vi "GetBroadcast.vi"(8 "Error In":errorcluster[](array[cluster]), 9 "BdcstInfo":variant, 11 "clBusData In":T2={"BusNumber"=0, "EvtPluginINIFilePath"=path "", "EvtParams"=[], "EvtConfig"={"UTC Time 0"=timestamp(0 s since 1904-01-01), "Nominal Frequency"=60, "Reporting Rate"=60, "Fsamp"=960, "PosSeq"=FALSE}, "Start Time"=0.0, "End Time"=0.0, "PmuImpairPluginINIFilePath"=path "", "PmuImpairParams "=[["960"], ["8.19"], ["164"]], "PmuImpairConfig"={"FilterType"="", "bPosSeq"=TRUE}, "NetImpPluginINIFilePath"=path "", "NetImpParams"=[], "FlagImpPluginINIFilePath"=path "", "FlagImpParams"=[], "EvtReportArray"=[], "EventSignalArray"=[], "ImpairReportArray"=[], "NetworkTime"=[], "PktLoss"=[], "FlagImpArray"=[], "OutputToFilePluginINIFilePath"=path "", "Output File Path"=path "", "clConfigOptions"={"TIME_BASE"=1000000, "STN"="Bus_1", "IDCODE"=0, "rdoPolRect"=enum."Rectangular", "rdoFloatInt"=enum."Float", "PHUNIT"=1000000, "rdoFreqDfreq"=enum."Float", "CHNAM"=["VA", "VB", "VC", "V+", "IA", "IB", "IC", "I+"], "chkCfg2Prefix"=TRUE}, "AppPluginINIFilePath"=path "", "AppConfig"=variant, "AppOutput"=variant} {"clConfigOptions"."PHUNIT" max=16777216 step=1 format="%08d"; "clConfigOptions"."IDCODE" format="%02x"; "clConfigOptions"."TIME_BASE" max=16777216 step=1 format="%08d"; "ImpairReportArray"."Synx" format="%#_4g"; "EvtReportArray"."Synx" format="%#_4g"; "EvtConfig"."Reporting Rate" items=["10 FPS"=10, "12 FPS"=12, "15 FPS"=15, "20 FPS"=20, "25 FPS"=25, "30 FPS"=30, "50 FPS"=50, "60 FPS"=60]; "EvtConfig"."Nominal Frequency" items=["50 Hz"=50, "60 Hz"=60]}) -> (0 "Error Out":errorcluster[](array[cluster]), 3 "clBusData Out":T2={"BusNumber"=0, "EvtPluginINIFilePath"=path "", "EvtParams"=[], "EvtConfig"={"UTC Time 0"=timestamp(0 s since 1904-01-01), "Nominal Frequency"=60, "Reporting Rate"=60, "Fsamp"=960, "PosSeq"=FALSE}, "Start Time"=0.0, "End Time"=0.0, "PmuImpairPluginINIFilePath"=path "", "PmuImpairParams "=[["960"], ["8.19"], ["164"]], "PmuImpairConfig"={"FilterType"="", "bPosSeq"=TRUE}, "NetImpPluginINIFilePath"=path "", "NetImpParams"=[], "FlagImpPluginINIFilePath"=path "", "FlagImpParams"=[], "EvtReportArray"=[], "EventSignalArray"=[], "ImpairReportArray"=[], "NetworkTime"=[], "PktLoss"=[], "FlagImpArray"=[], "OutputToFilePluginINIFilePath"=path "", "Output File Path"=path "", "clConfigOptions"={"TIME_BASE"=1000000, "STN"="Bus_1", "IDCODE"=0, "rdoPolRect"=enum."Rectangular", "rdoFloatInt"=enum."Float", "PHUNIT"=1000000, "rdoFreqDfreq"=enum."Float", "CHNAM"=["VA", "VB", "VC", "V+", "IA", "IB", "IC", "I+"], "chkCfg2Prefix"=TRUE}, "AppPluginINIFilePath"=path "", "AppConfig"=variant, "AppOutput"=variant} {"clConfigOptions"."PHUNIT" max=16777216 step=1 format="%08d"; "clConfigOptions"."IDCODE" format="%02x"; "clConfigOptions"."TIME_BASE" max=16777216 step=1 format="%08d"; "ImpairReportArray"."Synx" format="%#_4g"; "EvtReportArray"."Synx" format="%#_4g"; "EvtConfig"."Reporting Rate" items=["10 FPS"=10, "12 FPS"=12, "15 FPS"=15, "20 FPS"=20, "25 FPS"=25, "30 FPS"=30, "50 FPS"=50, "60 FPS"=60]; "EvtConfig"."Nominal Frequency" items=["50 Hz"=50, "60 Hz"=60]})   [LabVIEW 2017, in "Bus_class.lvlib" / "Bus.lvclass"]
uses:
  Bus.lvclass
  Public/TypeDefs/clBusData.ctl
  FrontPanel/TypeDefs/clEventConfig.ctl
  Modules/PmuImpairPlugins/PmuImpairPluginBase_class/TypeDefs/clImpairConfig.ctl
  Modules/EventPlugins/EventPluginBaseClass/TypeDefs/clEvtReportArray.ctl
  Modules/EventPlugins/EventPluginBaseClass/TypeDefs/clEvtReport.ctl
  Modules/EventPlugins/EventPluginBaseClass/TypeDefs/dblEvtSignalArray.ctl
  Modules/NetworkImpairmentModule/PublicAPI/Arguments/Broadcasts/dblNetworkTime.ctl
  Modules/NetworkImpairmentModule/PublicAPI/Arguments/Broadcasts/dblPktLoss.ctl
  Modules/FlagImpairModule/PublicAPI/Arguments/Broadcasts/ui32FlagImpairmentArray.ctl
  Modules/OutputToFilePlugins/OutputToFileBasePlugin/Typedefs/PmuCfgOpt.ctl
  ModuleType.ctl
  BdcstInfo.ctl
  Modules/EventModule/Protected/Broadcasts/clBroadcastEvents.ctl
  Modules/EventModule/Protected/clEventType.ctl
  Modules/EventModule/PublicAPI/Arguments/Broadcasts/clErrorRpt.ctl
  Modules/EventPlugins/EventPluginBaseClass/TypeDefs/clEvtConfig.ctl
  Modules/EventModule/PublicAPI/Arguments/Requests/dblTimeArray.ctl
  Modules/EventModule/PublicAPI/Arguments/Requests/dblEvtParams.ctl
  Modules/PmuImpairModule/Protected/Broadcasts/clBroadcastEvents.ctl
  Modules/PmuImpairModule/Protected/clEventType.ctl
  Modules/NetworkImpairmentModule/Protected/Broadcasts/clBroadcastEvents.ctl
  Modules/NetworkImpairmentModule/Protected/clEventType.ctl
  Modules/FlagImpairModule/Protected/Broadcasts/clBroadcastEvents.ctl
  Modules/FlagImpairModule/Protected/clEventType.ctl
  Modules/AppModule/Protected/Broadcasts/clBroadcastEvents.ctl
  Modules/AppModule/Protected/clEventType.ctl
  Modules/OutputToFileModule/Protected/Broadcasts/clBroadcastEvents.ctl
  Modules/OutputToFileModule/Private/clEventType.ctl
  <vilib>/Utility/error.llb/Error Cluster From Error Code.vi
  <vilib>/ErrorRing/Error Ring.xnode
  <userlib>/NIST/NISTErrorLib/NISTErrorLib.lvlib
  Modules/EventModule/EventModule.lvlib
  Framework.lvlib
  Modules/EventPlugins/EventPluginBaseClass/EventPluginBaseClass.lvclass
  Modules/PmuImpairPlugins/PmuImpairPluginBase_class/PmuImpairPluginBase.lvclass
  Modules/NetworkImpairmentModule/NetworkImpairmentModule.lvlib
  Modules/FlagImpairModule/FlagImpairModule.lvlib
  Modules/AppModule/AppModule.lvlib
  Modules/PmuImpairModule/PmuImpairModule.lvlib
  Modules/OutputToFileModule/OutputToFileModule.lvlib
  Modules/OutputToFilePlugins/OutputToFileBasePlugin/OutputToFileBasePlugin.lvclass
panel:
  out "ModuleType":T1
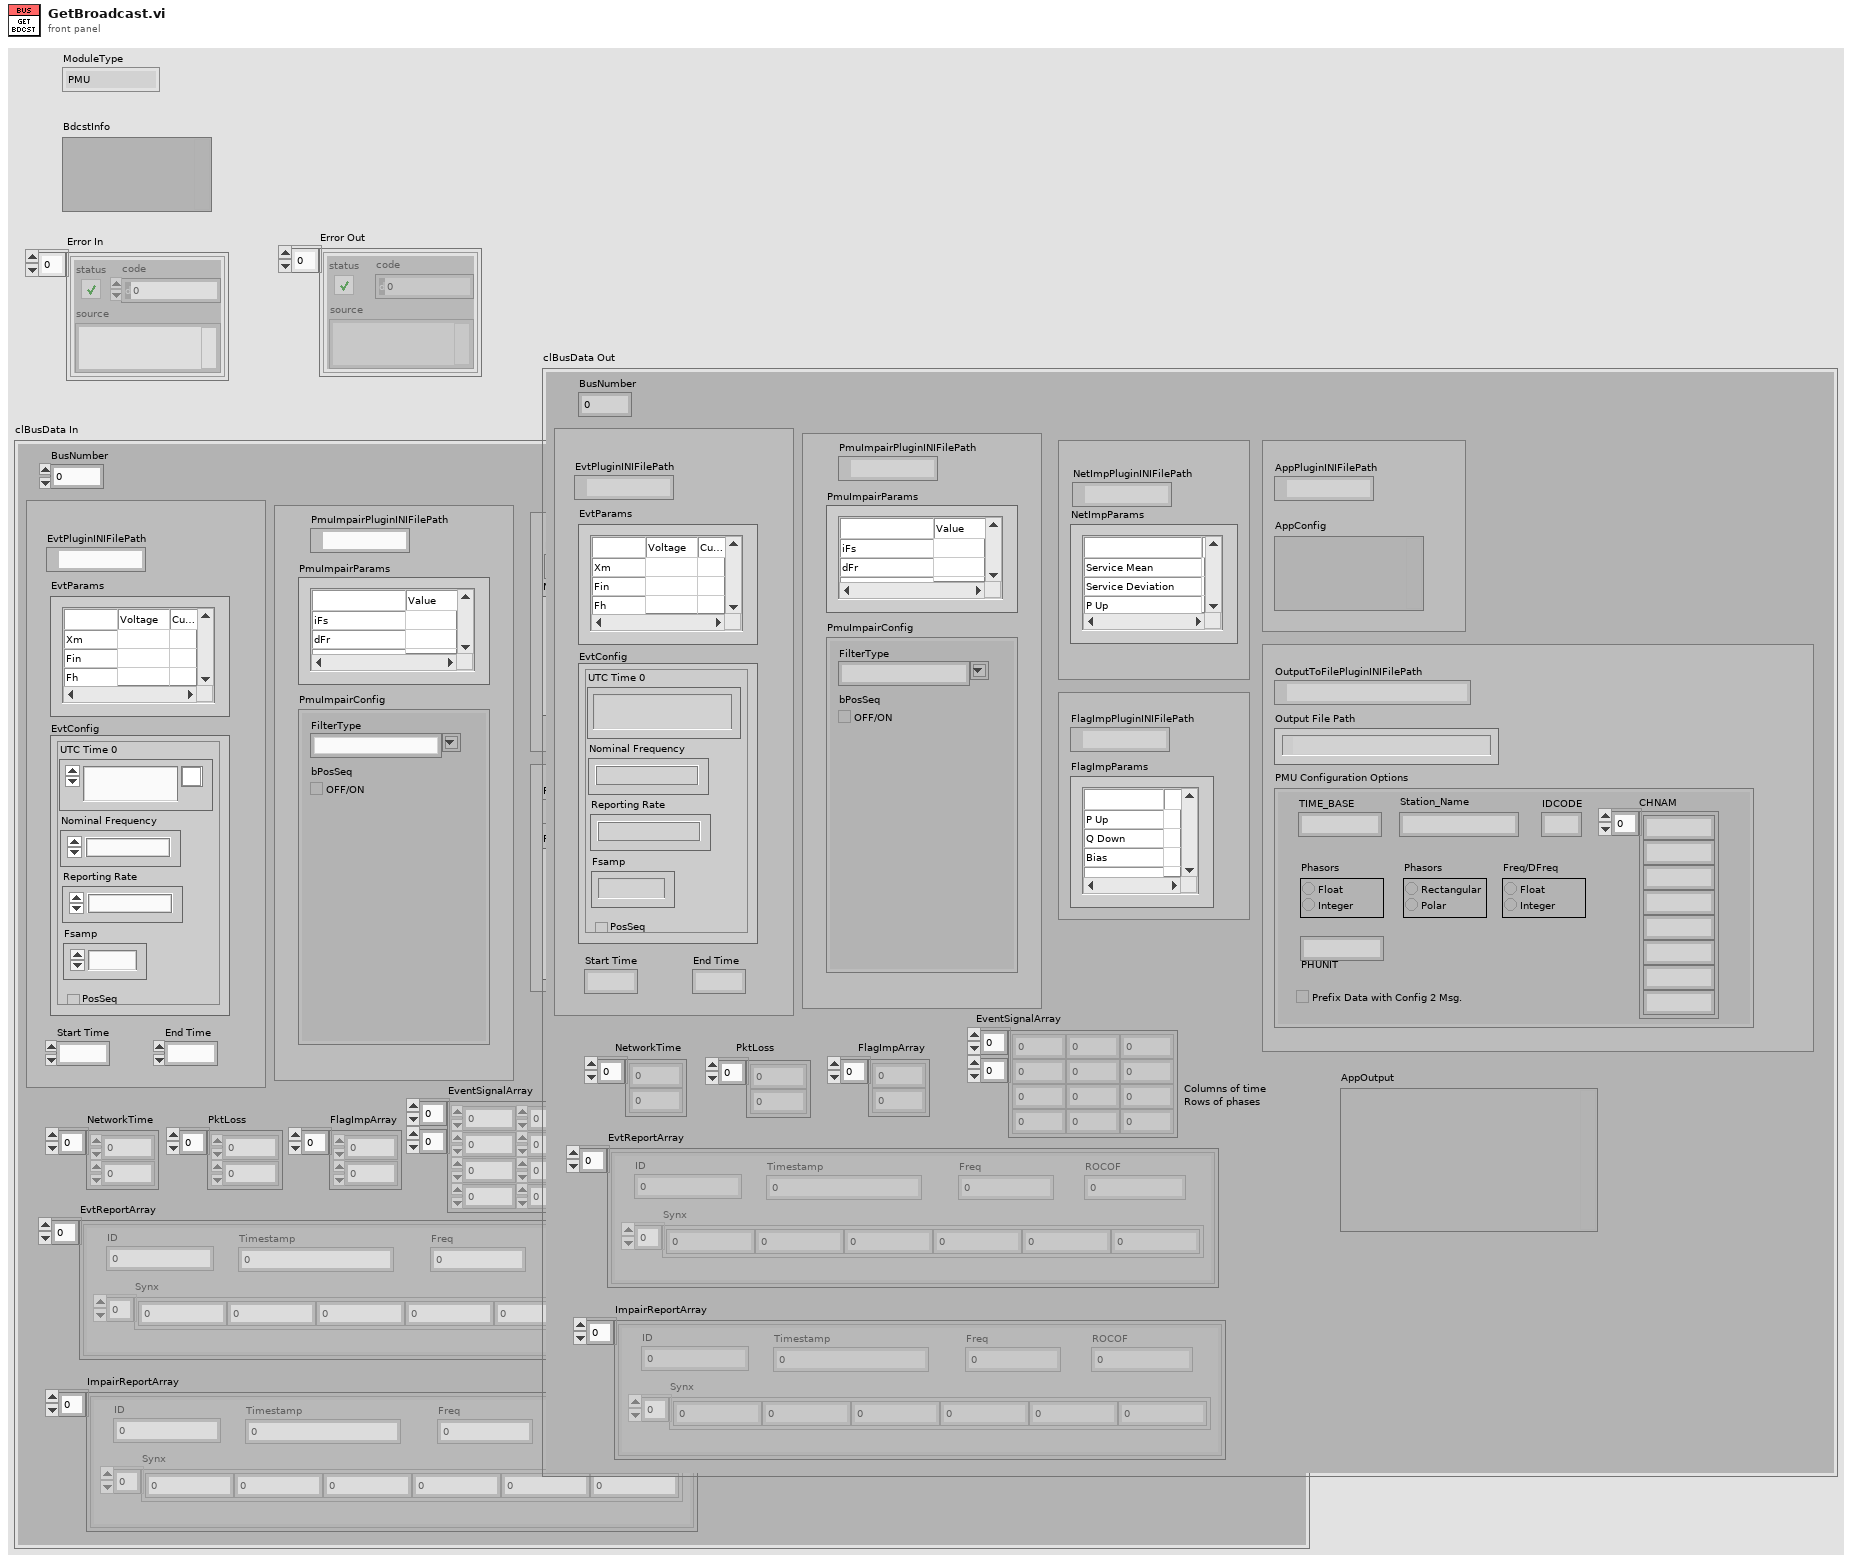
[diagram p1: front panel]
types:
  T1 = typedef "Bus_class.lvlib/Bus.lvclass/ModuleType.ctl" = enum16{"PMU", "Event", "Network", "Flag", "App", "OutToFile"}
  T2 = typedef "Bus_class.lvlib/Bus.lvclass/clBusData.ctl" = cluster{"BusNumber":u8, "EvtPluginINIFilePath":path, "EvtParams":string[][], "EvtConfig":T3, "Start Time":dbl, "End Time":dbl, "PmuImpairPluginINIFilePath":path, "PmuImpairParams ":string[][], "PmuImpairConfig":T4, "NetImpPluginINIFilePath":path, "NetImpParams":string[][], "FlagImpPluginINIFilePath":path, "FlagImpParams":string[][], "EvtReportArray":T5, "EventSignalArray":T7, "ImpairReportArray":T5, "NetworkTime":T8, "PktLoss":T9, "FlagImpArray":T10, "OutputToFilePluginINIFilePath":path, "Output File Path":path, "clConfigOptions":T11, "AppPluginINIFilePath":path, "AppConfig":variant, "AppOutput":variant}
  T3 = typedef "Framework.lvlib/clEventConfig.ctl" = cluster{"UTC Time 0":timestamp, "Nominal Frequency":u16, "Reporting Rate":u16, "Fsamp":u32, "PosSeq":bool}
  T4 = typedef "PmuImpairPlugins.lvlib/PmuImpairPluginBase.lvclass/clImpairConfig.ctl" = cluster{"FilterType":string, "bPosSeq":bool}
  T5 = typedef "EventPlugins.lvlib/EventPluginBaseClass.lvclass/clEvtReportArray.ctl" = T6[]
  T6 = typedef "EventPlugins.lvlib/EventPluginBaseClass.lvclass/clEvtReport.ctl" = cluster{"Timestamp":dbl, "Synx":cdb[], "Freq":dbl, "ROCOF":dbl, "ID":i16}
  T7 = typedef "EventPlugins.lvlib/EventPluginBaseClass.lvclass/dblEvtSignalArray.ctl" = dbl[][]
  T8 = typedef "NetworkImpairmentModule.lvlib/dblNetworkTime.ctl" = dbl[]
  T9 = typedef "NetworkImpairmentModule.lvlib/dblPktLoss.ctl" = dbl[]
  T10 = typedef "FlagImpairModule.lvlib/ui32FlagImpairmentArray.ctl" = u32[]
  T11 = typedef "OutputToFilePlugins.lvlib/OutputToFileBasePlugin.lvclass/PmuCfgOpt.ctl" = cluster{"TIME_BASE":u64, "STN":string, "IDCODE":u16, "rdoPolRect":enum32{"Rectangular", "Polar"}, "rdoFloatInt":enum32{"Float", "Integer"}, "PHUNIT":u64, "rdoFreqDfreq":enum32{"Float", "Integer"}, "CHNAM":string[], "chkCfg2Prefix":bool}
  T12 = typedef "Bus_class.lvlib/Bus.lvclass/BdcstInfo.ctl" = cluster{"ModuleType":T1, "ModuleID":i32, "UsrEvtRef":variant, "ScriptCmd":string}
  T13 = typedef "EventModule.lvlib/clErrorRpt.ctl" = cluster{"error":errorcluster, "AdditionalInfo":string}
  T14 = typedef "EventPlugins.lvlib/EventPluginBaseClass.lvclass/clEvtConfig.ctl" = cluster{"T0(UTC)":dbl, "F0":dbl, "Fs":i32, "FSamp":u32, "bPosSeq":bool}
  T15 = typedef "EventModule.lvlib/dblTimeArray.ctl" = dbl[]
  T16 = typedef "EventModule.lvlib/dblEvtParams.ctl" = dbl[][]
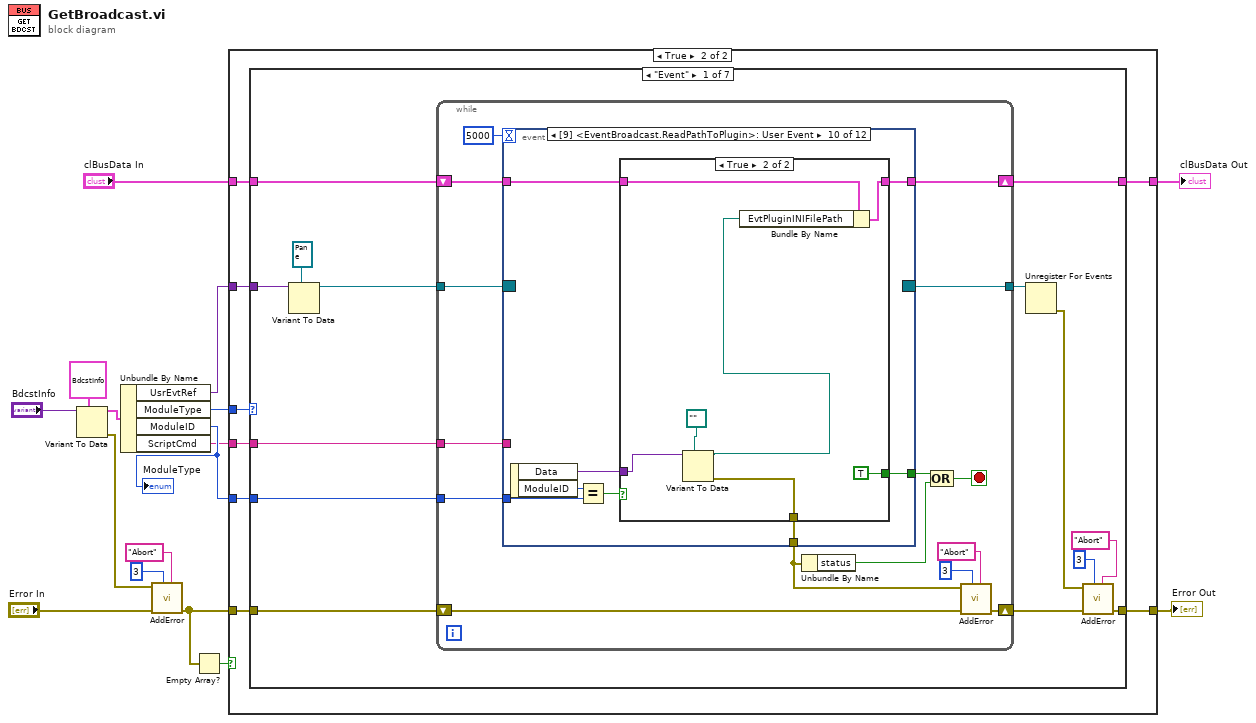
[diagram p0: block diagram]
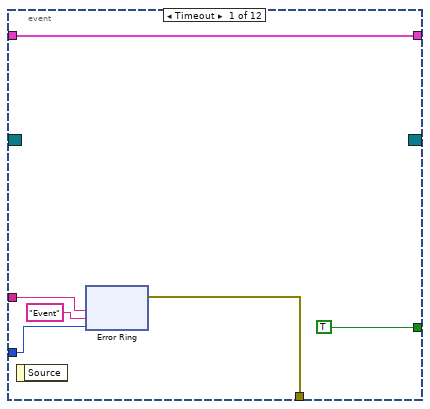
[diagram p3: hidden frame]
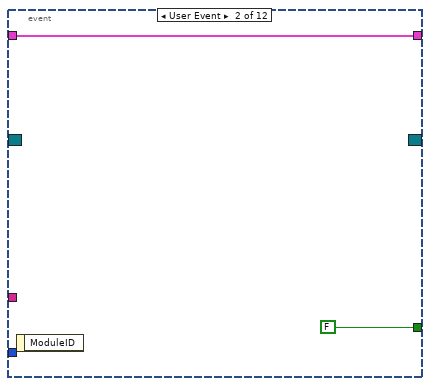
[diagram p4: hidden frame]
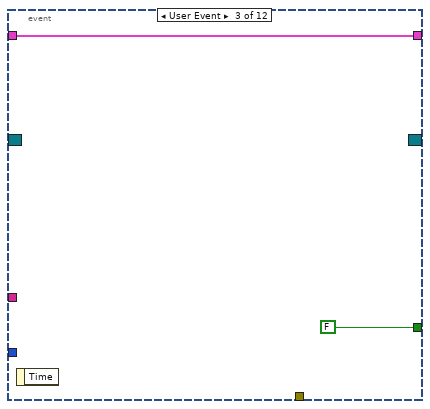
[diagram p5: hidden frame]
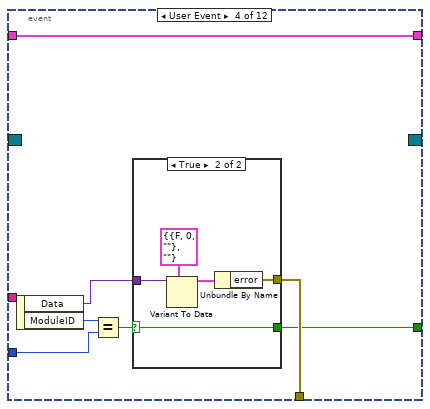
[diagram p6: hidden frame]
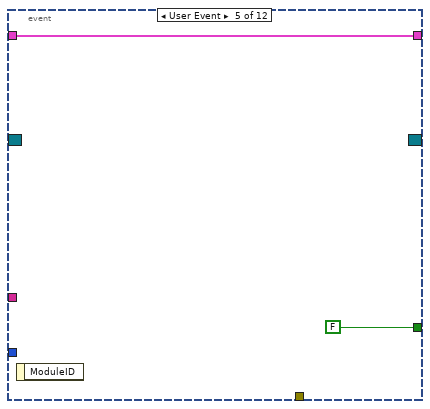
[diagram p8: hidden frame]
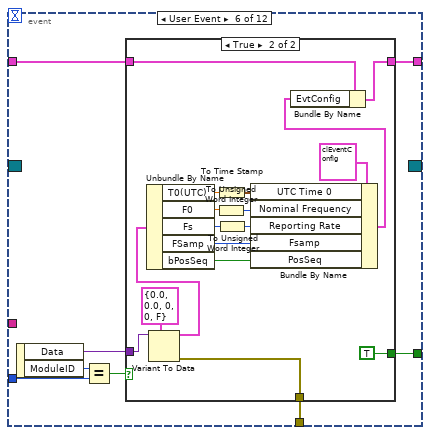
[diagram p9: hidden frame]
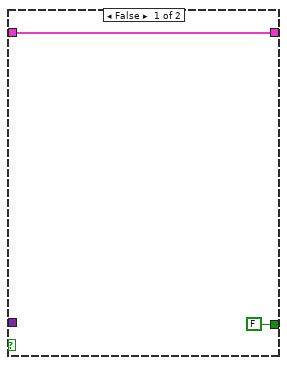
[diagram p10: hidden frame]
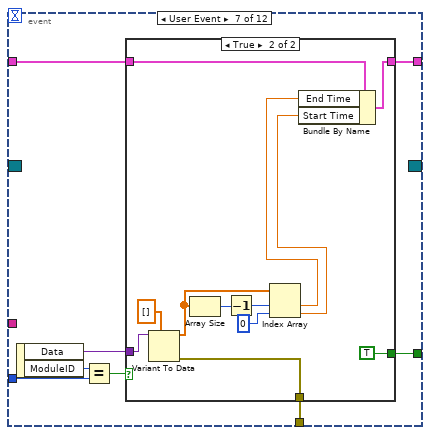
[diagram p11: hidden frame]
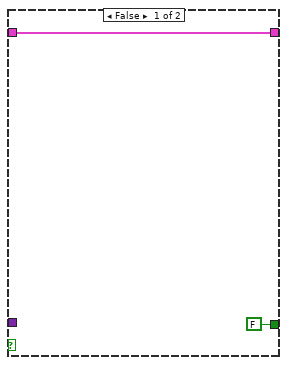
[diagram p12: hidden frame]
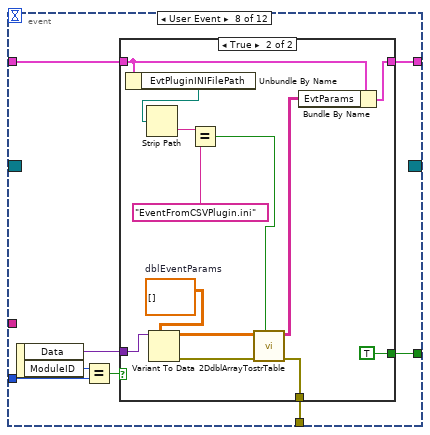
[diagram p13: hidden frame]
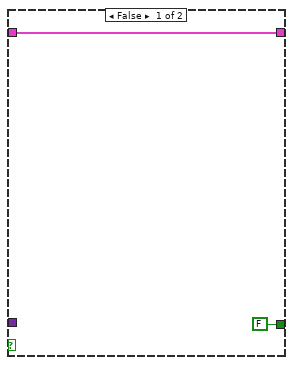
[diagram p14: hidden frame]
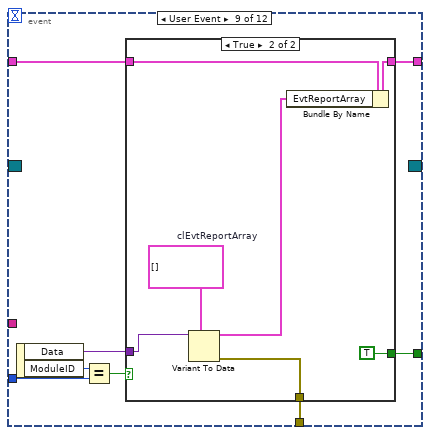
[diagram p15: hidden frame]
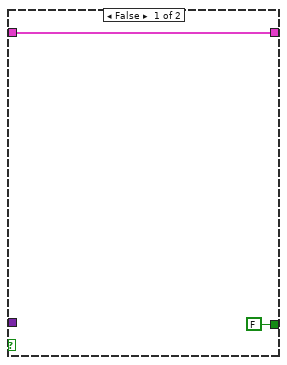
[diagram p16: hidden frame]
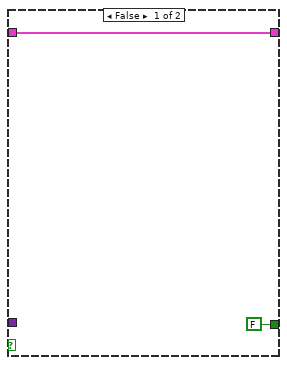
[diagram p17: hidden frame]
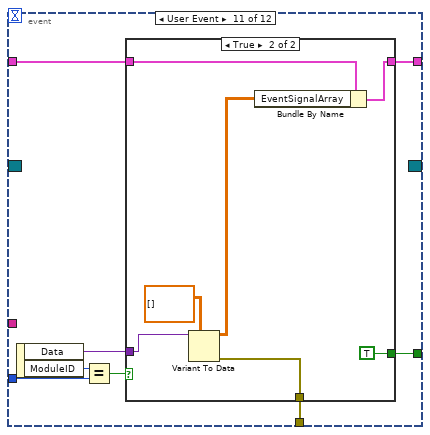
[diagram p18: hidden frame]
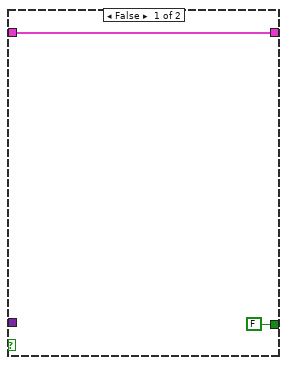
[diagram p19: hidden frame]
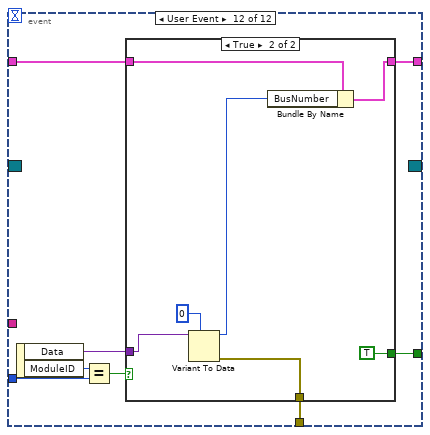
[diagram p20: hidden frame]
diagram:
  n1 = Variant To Data(type=T12 {"ModuleType"=enum."PMU", "ModuleID"=0, "UsrEvtRef"=variant, "ScriptCmd"=""} ("BdcstInfo"), Variant="BdcstInfo") -> (data=w10:T12, error out=w5:errorcluster)  [unwired: 1 in]
  n2 = Unbundle By Name(w10) -> ("UsrEvtRef"=w8:variant, "ModuleType"=w9:T1, "ModuleID"=w2:i32, "ScriptCmd"=w1:string)
  "ModuleType" <- w2
  n3 = call <userlib>:"AddError.vi"("Severity"="Abort", "Priority"=u8 3, "ErrorArray"="Error In", "error in (no error)"=w5) -> ("ErrorArray"=w7:errorcluster[])  [unwired: 6 in, 1 out]
  n4 = Empty Array?(array=w7) -> (empty?=w16:bool)
  n5 = case shown="True" w16 {
    tunnel: [w18 w24] -> w15
    tunnel: w7 -> [w18 w25]
    tunnel: w9 -> [_ w26]
    tunnel: w2 -> [_ w23]
    tunnel: "clBusData In" -> [w17 w22]
    tunnel: [w17 w21] -> w13
    tunnel: w8 -> [_ w20]
    tunnel: w1 -> [_ w19]
    frame False {
    }
    frame True {
      n6 = case shown="\"Event\"" w26 {
        tunnel: w25 -> [w40 w242 w391 w533 w653 w793 w910]
        tunnel: [w30 w232 w382 w527 w660 w800 w908] -> w24
        tunnel: w23 -> [w38 w240 w389 w531 w664 w804 _]
        tunnel: w22 -> [w37 w239 w388 w530 w663 w803 w905]
        tunnel: [w36 w238 w387 w529 w662 w802 w905] -> w21
        tunnel: w20 -> [w35 w236 w385 w522 w649 w790 _]
        tunnel: w19 -> [w32 w237 w386 w523 w652 w792 _]
        frame "Event" {
          n7 = Variant To Data(type=refnum<event-registration> refnum ("event registration refnum"), Variant=w35) -> (data=w33:refnum<event-registration>)  [unwired: 1 in, 1 out]
          n8 = while {
            tunnel: w38 -> [w54]
            tunnel: w33 -> [w53]
            shift-right: [w51] -> w31
            shift-left: w40 -> [w52]
            tunnel: [w46] -> w39
            shift-right: [w44] -> w36
            shift-left: w37 -> [w45]
            tunnel: w32 -> [w41]
            stop <- w47 stop-if-true
            n9 = event shown="[9] <EventBroadcast.ReadPathToPlugin>: User Event" {
              selector: w53 -> [_ _ _ _ _ _ _ _ _ _ _ _]
              dyn-events: [_ _ _ _ _ _ _ _ _ _ _ _] -> w46
              timeout: 5000 -> [_ _ _ _ _ _ _ _ _ _ _ _]
              tunnel: w54 -> [w58 _ _ w81 _ w96 w123 w145 w167 w184 w201 w218]
              tunnel: [w61 _ _ w78 _ w90 w117 w139 w161 w178 w195 w212] -> w50
              tunnel: [TRUE FALSE FALSE w76 FALSE w94 w121 w143 w165 w182 w199 w216] -> w49
              tunnel: w45 -> [w59 w71 w73 w75 w88 w92 w119 w141 w163 w180 w197 w214]
              tunnel: [w59 w71 w73 w75 w88 w91 w118 w140 w162 w179 w196 w213] -> w44
              tunnel: w41 -> [w56 _ _ _ _ _ _ _ _ _ _ _]
              event Timeout {
                n10 = event-data() -> ()  [unwired: 1 in, 1 out]
                n11 = xnode "Error Ring"("parameter 0"=w56, "parameter 1"="Event" ("parameter 0"), "parameter 2"=w58) -> ("error out"=w61:errorcluster)
              }
              event User Event {
                n12 = event-data() -> ()  [unwired: 1 in, 1 out]
              }
              event User Event {
                n13 = event-data() -> ()  [unwired: 1 in, 1 out]
              }
              event User Event {
                n14 = event-data() -> ("Data"=w79:variant, "ModuleID"=w80:i32)  [unwired: 1 in]
                n15 = Equal?(x=w80, y=w81) -> (x = y?=w77:bool)
                n16 = case shown="True" w77 {
                  selector: w77 -> [w82 w83]
                  tunnel: w79 -> [_ w87]
                  tunnel: [_ w84] -> w78
                  tunnel: [w82 w83] -> w76
                  frame False {
                  }
                  frame True {
                    n17 = Variant To Data(type=T13 {"error"={"status"=FALSE, "code"=0, "source"=""}, "AdditionalInfo"=""} ("Cluster"), Variant=w87) -> (data=w85:T13)  [unwired: 1 in, 1 out]
                    n18 = Unbundle By Name(w85) -> ("error"=w84:errorcluster)
                  }
                }
              }
              event User Event {
                n19 = event-data() -> ()  [unwired: 1 in, 1 out]
              }
              event User Event {
                n20 = event-data() -> ("Data"=w93:variant, "ModuleID"=w97:i32)  [unwired: 1 in]
                n21 = Equal?(x=w97, y=w96) -> (x = y?=w95:bool)
                n22 = case shown="True" w95 {
                  tunnel: [FALSE TRUE] -> w94
                  tunnel: w93 -> [_ w116]
                  tunnel: w92 -> [w98 w103]
                  tunnel: [w98 w101] -> w91
                  tunnel: [_ w100] -> w90
                  frame False {
                  }
                  frame True {
                    n23 = Variant To Data(type=T14 {"T0(UTC)"=0.0, "F0"=0.0, "Fs"=0, "FSamp"=0, "bPosSeq"=FALSE} ("clEvtConfig"), Variant=w116) -> (data=w105:T14, error out=w100:errorcluster)  [unwired: 1 in]
                    n24 = Unbundle By Name(w105) -> ("T0(UTC)"=w113:dbl, "F0"=w111:dbl, "Fs"=w108:i32, "FSamp"=w107:u32, "bPosSeq"=w115:bool)
                    n25 = To Unsigned Word Integer(number=w111) -> (unsigned 16bit integer=w110:u16)
                    n26 = To Time Stamp(1:w113) -> (0:w112:timestamp)
                    n27 = To Unsigned Word Integer(number=w108) -> (unsigned 16bit integer=w109:u16)
                    n28 = Bundle By Name(cluster=T3 {"UTC Time 0"=timestamp(0 s since 1904-01-01), "Nominal Frequency"=60, "Reporting Rate"=60, "Fsamp"=960, "PosSeq"=FALSE} ("Event Configuration 2"), "UTC Time 0"=w112, "Nominal Frequency"=w110, "Reporting Rate"=w109, "Fsamp"=w107, "PosSeq"=w115) -> (w102:T3)
                    n29 = Bundle By Name(cluster=w103, "EvtConfig"=w102) -> (w101:T2)
                  }
                }
              }
              event User Event {
                n30 = event-data() -> ("Data"=w120:variant, "ModuleID"=w124:i32)  [unwired: 1 in]
                n31 = Equal?(x=w124, y=w123) -> (x = y?=w122:bool)
                n32 = case shown="True" w122 {
                  tunnel: [FALSE TRUE] -> w121
                  tunnel: w120 -> [_ w138]
                  tunnel: w119 -> [w125 w136]
                  tunnel: [w125 w135] -> w118
                  tunnel: [_ w127] -> w117
                  frame False {
                  }
                  frame True {
                    n33 = Variant To Data(type=T15 [] ("dblTimeArray"), Variant=w138) -> (data=w130:T15, error out=w127:errorcluster)  [unwired: 1 in]
                    n34 = Array Size(array=w130) -> (size(s)=w131:i32)
                    n35 = Decrement(x=w131) -> (x-1=w132:i32)
                    n36 = Index Array(array=w130, index #1=w132, index #2=0 ("index")) -> (element #1=w129:dbl, element #2=w128:dbl)
                    n37 = Bundle By Name(cluster=w136, "End Time"=w129, "Start Time"=w128) -> (w135:T2)
                  }
                }
              }
              event User Event {
                n38 = event-data() -> ("Data"=w142:variant, "ModuleID"=w146:i32)  [unwired: 1 in]
                n39 = Equal?(x=w146, y=w145) -> (x = y?=w144:bool)
                n40 = case shown="True" w144 {
                  tunnel: [FALSE TRUE] -> w143
                  tunnel: w142 -> [_ w160]
                  tunnel: w141 -> [w147 w153]
                  tunnel: [w147 w158] -> w140
                  tunnel: [_ w154] -> w139
                  frame False {
                  }
                  frame True {
                    w157 = T16 []  # dblEventParams
                    n41 = Unbundle By Name(w153) -> ("EvtPluginINIFilePath"=w152:path)
                    n42 = Strip Path(path=w152) -> (name=w151:string)  [unwired: 1 out]
                    n43 = Variant To Data(type=w157, Variant=w160) -> (data=w156:T16, error out=w154:errorcluster)  [unwired: 1 in]
                    n44 = Equal?(x=w151, y="EventFromCSVPlugin.ini") -> (x = y?=w149:bool)
                    n45 = call "2DdblArrayTostrTable.vi"("RowsAreStrings (f)"=w149, "dbl2DArray"=w156) -> ("strTable"=w155:string[][])  [unwired: 9 in]
                    n46 = Bundle By Name(cluster=w153, "EvtParams"=w155) -> (w158:T2)
                  }
                }
              }
              event User Event {
                n47 = event-data() -> ("Data"=w164:variant, "ModuleID"=w168:i32)  [unwired: 1 in]
                n48 = Equal?(x=w168, y=w167) -> (x = y?=w166:bool)
                n49 = case shown="True" w166 {
                  tunnel: [FALSE TRUE] -> w165
                  tunnel: w164 -> [_ w177]
                  tunnel: w163 -> [w169 w175]
                  tunnel: [w169 w174] -> w162
                  tunnel: [_ w171] -> w161
                  frame False {
                  }
                  frame True {
                    w173 = T5 []  # clEvtReportArray
                    n50 = Variant To Data(type=w173, Variant=w177) -> (data=w172:T5, error out=w171:errorcluster)  [unwired: 1 in]
                    n51 = Bundle By Name(cluster=w175, "EvtReportArray"=w172) -> (w174:T2)
                  }
                }
              }
              event User Event {
                n52 = event-data() -> ("Data"=w181:variant, "ModuleID"=w185:i32)  [unwired: 1 in]
                n53 = Equal?(x=w185, y=w184) -> (x = y?=w183:bool)
                n54 = case shown="True" w183 {
                  tunnel: [FALSE TRUE] -> w182
                  tunnel: w181 -> [_ w194]
                  tunnel: w180 -> [w186 w192]
                  tunnel: [w186 w191] -> w179
                  tunnel: [_ w190] -> w178
                  frame False {
                  }
                  frame True {
                    n55 = Variant To Data(type=path "", Variant=w194) -> (data=w188:path, error out=w190:errorcluster)  [unwired: 1 in]
                    n56 = Bundle By Name(cluster=w192, "EvtPluginINIFilePath"=w188) -> (w191:T2)
                  }
                }
              }
              event User Event {
                n57 = event-data() -> ("Data"=w198:variant, "ModuleID"=w202:i32)  [unwired: 1 in]
                n58 = Equal?(x=w202, y=w201) -> (x = y?=w200:bool)
                n59 = case shown="True" w200 {
                  tunnel: [FALSE TRUE] -> w199
                  tunnel: w198 -> [_ w211]
                  tunnel: w197 -> [w203 w209]
                  tunnel: [w203 w208] -> w196
                  tunnel: [_ w207] -> w195
                  frame False {
                  }
                  frame True {
                    n60 = Variant To Data(type=T7 [] ("dblEventSignalArray"), Variant=w211) -> (data=w205:T7, error out=w207:errorcluster)  [unwired: 1 in]
                    n61 = Bundle By Name(cluster=w209, "EventSignalArray"=w205) -> (w208:T2)
                  }
                }
              }
              event User Event {
                n62 = event-data() -> ("Data"=w215:variant, "ModuleID"=w219:i32)  [unwired: 1 in]
                n63 = Equal?(x=w219, y=w218) -> (x = y?=w217:bool)
                n64 = case shown="True" w217 {
                  tunnel: [FALSE TRUE] -> w216
                  tunnel: w215 -> [_ w228]
                  tunnel: w214 -> [w220 w226]
                  tunnel: [w220 w225] -> w213
                  tunnel: [_ w224] -> w212
                  frame False {
                  }
                  frame True {
                    n65 = Variant To Data(type=u8 0 ("BusNumber"), Variant=w228) -> (data=w222:u8, error out=w224:errorcluster)  [unwired: 1 in]
                    n66 = Bundle By Name(cluster=w226, "BusNumber"=w222) -> (w225:T2)
                  }
                }
              }
            }
            n67 = Unbundle By Name(w50) -> ("status"=w48:bool)
            n68 = Compound Arithmetic op=OR(w49, w48) -> (w47:bool)
            n69 = call <userlib>:"AddError.vi"("Severity"="Abort", "Priority"=u8 3, "ErrorArray"=w52, "error in (no error)"=w50) -> ("ErrorArray"=w51:errorcluster[])  [unwired: 6 in, 1 out]
          }
          n70 = Unregister For Events(event registration refnum=w39) -> (error out=w29:errorcluster)  [unwired: 1 in]
          n71 = call <userlib>:"AddError.vi"("Severity"="Abort", "Priority"=u8 3, "ErrorArray"=w31, "error in (no error)"=w29) -> ("ErrorArray"=w30:errorcluster[])  [unwired: 6 in, 1 out]
        }
        frame "PMU" {
          n72 = Variant To Data(type=refnum<event-registration> refnum ("event registration refnum"), Variant=w236) -> (data=w235:refnum<event-registration>)  [unwired: 1 in, 1 out]
          n73 = while {
            tunnel: w240 -> [w256]
            tunnel: w235 -> [w255]
            shift-right: [w253] -> w233
            shift-left: w242 -> [w254]
            tunnel: [w248] -> w241
            shift-right: [w246] -> w238
            shift-left: w239 -> [w247]
            tunnel: w237 -> [w243]
            stop <- w249 stop-if-true
            n74 = event shown="[8] <ImpairBroadcast.PathToPlugin>: User Event" {
              selector: w255 -> [_ _ _ _ _ _ _ _ _ _]
              dyn-events: [_ _ _ _ _ _ _ _ _ _] -> w248
              timeout: 5000 -> [_ _ _ _ _ _ _ _ _ _]
              tunnel: w256 -> [w261 _ _ w283 _ w298 w315 w333 w350 w367]
              tunnel: [w258 _ _ w280 _ w292 w309 w327 w344 w361] -> w252
              tunnel: [TRUE FALSE FALSE w278 FALSE w296 w313 w331 w348 w365] -> w251
              tunnel: w247 -> [w262 w273 w275 w277 w290 w294 w311 w329 w346 w363]
              tunnel: [w262 w273 w275 w277 w290 w293 w310 w328 w345 w362] -> w246
              tunnel: w243 -> [w259 _ _ _ _ _ _ _ _ _]
              event Timeout {
                n75 = event-data() -> ()  [unwired: 1 in, 1 out]
                n76 = xnode "Error Ring"("parameter 0"=w259, "parameter 1"="PMU" ("parameter 0"), "parameter 2"=w261) -> ("error out"=w258:errorcluster)
              }
              event User Event {
                n77 = event-data() -> ()  [unwired: 1 in, 1 out]
              }
              event User Event {
                n78 = event-data() -> ()  [unwired: 1 in, 1 out]
              }
              event User Event {
                n79 = event-data() -> ("Data"=w281:variant, "ModuleID"=w282:i32)  [unwired: 1 in]
                n80 = Equal?(x=w282, y=w283) -> (x = y?=w279:bool)
                n81 = case shown="True" w279 {
                  selector: w279 -> [w284 w285]
                  tunnel: w281 -> [_ w289]
                  tunnel: [_ w286] -> w280
                  tunnel: [w284 w285] -> w278
                  frame False {
                  }
                  frame True {
                    n82 = Variant To Data(type=T13 {"error"={"status"=FALSE, "code"=0, "source"=""}, "AdditionalInfo"=""} ("Cluster"), Variant=w289) -> (data=w287:T13)  [unwired: 1 in, 1 out]
                    n83 = Unbundle By Name(w287) -> ("error"=w286:errorcluster)
                  }
                }
              }
              event User Event {
                n84 = event-data() -> ()  [unwired: 1 in, 1 out]
              }
              event User Event {
                n85 = event-data() -> ("Data"=w295:variant, "ModuleID"=w299:i32)  [unwired: 1 in]
                n86 = Equal?(x=w299, y=w298) -> (x = y?=w297:bool)
                n87 = case shown="True" w297 {
                  tunnel: [FALSE TRUE] -> w296
                  tunnel: w295 -> [_ w308]
                  tunnel: w294 -> [w300 w306]
                  tunnel: [w300 w305] -> w293
                  tunnel: [_ w302] -> w292
                  frame False {
                  }
                  frame True {
                    n88 = Variant To Data(type=T4 {"FilterType"="", "bPosSeq"=TRUE} ("clImpairConfig"), Variant=w308) -> (data=w303:T4, error out=w302:errorcluster)  [unwired: 1 in]
                    n89 = Bundle By Name(cluster=w306, "PmuImpairConfig"=w303) -> (w305:T2)
                  }
                }
              }
              event User Event {
                n90 = event-data() -> ("Data"=w312:variant, "ModuleID"=w316:i32)  [unwired: 1 in]
                n91 = Equal?(x=w316, y=w315) -> (x = y?=w314:bool)
                n92 = case shown="True" w314 {
                  tunnel: [FALSE TRUE] -> w313
                  tunnel: w312 -> [_ w326]
                  tunnel: w311 -> [w317 w324]
                  tunnel: [w317 w323] -> w310
                  tunnel: [_ w319] -> w309
                  frame False {
                  }
                  frame True {
                    n93 = Variant To Data(type=T16 [] ("dblEventParams"), Variant=w326) -> (data=w321:T16, error out=w319:errorcluster)  [unwired: 1 in]
                    n94 = call "2DdblArrayTostrTable.vi"("dbl2DArray"=w321) -> ("strTable"=w320:string[][])  [unwired: 10 in]
                    n95 = Bundle By Name(cluster=w324, "PmuImpairParams"=w320) -> (w323:T2)
                  }
                }
              }
              event User Event {
                n96 = event-data() -> ("Data"=w330:variant, "ModuleID"=w334:i32)  [unwired: 1 in]
                n97 = Equal?(x=w334, y=w333) -> (x = y?=w332:bool)
                n98 = case shown="True" w332 {
                  tunnel: [FALSE TRUE] -> w331
                  tunnel: w330 -> [_ w343]
                  tunnel: w329 -> [w335 w341]
                  tunnel: [w335 w340] -> w328
                  tunnel: [_ w337] -> w327
                  frame False {
                  }
                  frame True {
                    w339 = T5 []  # clEvtReportArray
                    n99 = Variant To Data(type=w339, Variant=w343) -> (data=w338:T5, error out=w337:errorcluster)  [unwired: 1 in]
                    n100 = Bundle By Name(cluster=w341, "ImpairReportArray"=w338) -> (w340:T2)
                  }
                }
              }
              event User Event {
                n101 = event-data() -> ("Data"=w347:variant, "ModuleID"=w351:i32)  [unwired: 1 in]
                n102 = Equal?(x=w351, y=w350) -> (x = y?=w349:bool)
                n103 = case shown="True" w349 {
                  tunnel: [FALSE TRUE] -> w348
                  tunnel: w347 -> [_ w360]
                  tunnel: w346 -> [w352 w358]
                  tunnel: [w352 w357] -> w345
                  tunnel: [_ w356] -> w344
                  frame False {
                  }
                  frame True {
                    n104 = Variant To Data(type=path "", Variant=w360) -> (data=w354:path, error out=w356:errorcluster)  [unwired: 1 in]
                    n105 = Bundle By Name(cluster=w358, "PmuImpairPluginINIFilePath"=w354) -> (w357:T2)
                  }
                }
              }
              event User Event {
                n106 = event-data() -> ("Data"=w364:variant, "ModuleID"=w368:i32)  [unwired: 1 in]
                n107 = Equal?(x=w368, y=w367) -> (x = y?=w366:bool)
                n108 = case shown="True" w366 {
                  tunnel: [FALSE TRUE] -> w365
                  tunnel: w364 -> [_ w377]
                  tunnel: w363 -> [w369 w375]
                  tunnel: [w369 w374] -> w362
                  tunnel: [_ w373] -> w361
                  frame False {
                  }
                  frame True {
                    n109 = Variant To Data(type=u8 0 ("BusNumber"), Variant=w377) -> (data=w371:u8, error out=w373:errorcluster)  [unwired: 1 in]
                    n110 = Bundle By Name(cluster=w375, "BusNumber"=w371) -> (w374:T2)
                  }
                }
              }
            }
            n111 = Unbundle By Name(w252) -> ("status"=w250:bool)
            n112 = Compound Arithmetic op=OR(w251, w250) -> (w249:bool)
            n113 = call <userlib>:"AddError.vi"("Severity"="Abort", "Priority"=u8 3, "ErrorArray"=w254, "error in (no error)"=w252) -> ("ErrorArray"=w253:errorcluster[])  [unwired: 6 in, 1 out]
          }
          n114 = Unregister For Events(event registration refnum=w241) -> (error out=w231:errorcluster)  [unwired: 1 in]
          n115 = call <userlib>:"AddError.vi"("Severity"="Abort", "Priority"=u8 3, "ErrorArray"=w233, "error in (no error)"=w231) -> ("ErrorArray"=w232:errorcluster[])  [unwired: 6 in, 1 out]
        }
        frame "Network" {
          n116 = Variant To Data(type=refnum<event-registration> refnum ("Event Registration Refnum"), Variant=w385) -> (data=w383:refnum<event-registration>)  [unwired: 1 in, 1 out]
          n117 = while {
            tunnel: w389 -> [w405]
            tunnel: w383 -> [w404]
            shift-right: [w402] -> w381
            shift-left: w391 -> [w403]
            tunnel: [w397] -> w390
            shift-right: [w395] -> w387
            shift-left: w388 -> [w396]
            tunnel: w386 -> [w392]
            stop <- w398 stop-if-true
            n118 = event shown="[8] <NetImpBroadcast.ReadPathToPlugin>: User Event" {
              selector: w404 -> [_ _ _ _ _ _ _ _ _ _]
              dyn-events: [_ _ _ _ _ _ _ _ _ _] -> w397
              timeout: 5000 -> [_ _ _ _ _ _ _ _ _ _]
              tunnel: w405 -> [w409 _ _ w432 _ w444 w457 w475 w492 w509]
              tunnel: [w410 _ _ w429 _ _ w451 w469 w486 w503] -> w401
              tunnel: [TRUE FALSE FALSE w427 FALSE w446 w455 w473 w490 w507] -> w400
              tunnel: w396 -> [w411 w422 w424 w426 w439 w442 w453 w471 w488 w505]
              tunnel: [w411 w422 w424 w426 w439 w441 w452 w470 w487 w504] -> w395
              tunnel: w392 -> [w407 _ _ _ _ _ _ _ _ _]
              event Timeout {
                n119 = event-data() -> ()  [unwired: 1 in, 1 out]
                n120 = xnode "Error Ring"("parameter 0"=w407, "parameter 1"="Network" ("parameter 0"), "parameter 2"=w409) -> ("error out"=w410:errorcluster)
              }
              event User Event {
                n121 = event-data() -> ()  [unwired: 1 in, 1 out]
              }
              event User Event {
                n122 = event-data() -> ()  [unwired: 1 in, 1 out]
              }
              event User Event {
                n123 = event-data() -> ("Data"=w430:variant, "ModuleID"=w431:i32)  [unwired: 1 in]
                n124 = Equal?(x=w431, y=w432) -> (x = y?=w428:bool)
                n125 = case shown="True" w428 {
                  selector: w428 -> [w433 w434]
                  tunnel: w430 -> [_ w438]
                  tunnel: [_ w435] -> w429
                  tunnel: [w433 w434] -> w427
                  frame False {
                  }
                  frame True {
                    n126 = Variant To Data(type=T13 {"error"={"status"=FALSE, "code"=0, "source"=""}, "AdditionalInfo"=""} ("Cluster"), Variant=w438) -> (data=w436:T13)  [unwired: 1 in, 1 out]
                    n127 = Unbundle By Name(w436) -> ("error"=w435:errorcluster)
                  }
                }
              }
              event User Event {
                n128 = event-data() -> ()  [unwired: 1 in, 1 out]
              }
              event User Event {
                n129 = event-data() -> ("ModuleID"=w445:i32)  [unwired: 1 in, 1 out]
                n130 = Equal?(x=w445, y=w444) -> (x = y?=w443:bool)
                n131 = case shown="True" w443 {
                  tunnel: [FALSE TRUE] -> w446
                  tunnel: [w447 w449] -> w441
                  tunnel: w442 -> [w447 w449]
                  frame False {
                  }
                  frame True {
                  }
                }
              }
              event User Event {
                n132 = event-data() -> ("Data"=w454:variant, "ModuleID"=w458:i32)  [unwired: 1 in]
                n133 = Equal?(x=w458, y=w457) -> (x = y?=w456:bool)
                n134 = case shown="True" w456 {
                  tunnel: [FALSE TRUE] -> w455
                  tunnel: w454 -> [_ w468]
                  tunnel: w453 -> [w459 w466]
                  tunnel: [w459 w465] -> w452
                  tunnel: [_ w461] -> w451
                  frame False {
                  }
                  frame True {
                    n135 = Variant To Data(type=T16 [] ("dblEventParams"), Variant=w468) -> (data=w463:T16, error out=w461:errorcluster)  [unwired: 1 in]
                    n136 = call "2DdblArrayTostrTable.vi"("dbl2DArray"=w463) -> ("strTable"=w462:string[][])  [unwired: 10 in]
                    n137 = Bundle By Name(cluster=w466, "NetImpParams"=w462) -> (w465:T2)
                  }
                }
              }
              event User Event {
                n138 = event-data() -> ("Data"=w472:variant, "ModuleID"=w476:i32)  [unwired: 1 in]
                n139 = Equal?(x=w476, y=w475) -> (x = y?=w474:bool)
                n140 = case shown="True" w474 {
                  tunnel: [FALSE TRUE] -> w473
                  tunnel: w472 -> [_ w485]
                  tunnel: w471 -> [w477 w483]
                  tunnel: [w477 w482] -> w470
                  tunnel: [_ w480] -> w469
                  frame False {
                  }
                  frame True {
                    w479 = T9 []  # dblPktLoss
                    n141 = Variant To Data(type=w479, Variant=w485) -> (data=w481:T9, error out=w480:errorcluster)  [unwired: 1 in]
                    n142 = Bundle By Name(cluster=w483, "PktLoss"=w481) -> (w482:T2)
                  }
                }
              }
              event User Event {
                n143 = event-data() -> ("Data"=w489:variant, "ModuleID"=w493:i32)  [unwired: 1 in]
                n144 = Equal?(x=w493, y=w492) -> (x = y?=w491:bool)
                n145 = case shown="True" w491 {
                  tunnel: [FALSE TRUE] -> w490
                  tunnel: w489 -> [_ w502]
                  tunnel: w488 -> [w494 w500]
                  tunnel: [w494 w499] -> w487
                  tunnel: [_ w498] -> w486
                  frame False {
                  }
                  frame True {
                    n146 = Variant To Data(type=path "", Variant=w502) -> (data=w496:path, error out=w498:errorcluster)  [unwired: 1 in]
                    n147 = Bundle By Name(cluster=w500, "NetImpPluginINIFilePath"=w496) -> (w499:T2)
                  }
                }
              }
              event User Event {
                n148 = event-data() -> ("Data"=w506:variant, "ModuleID"=w510:i32)  [unwired: 1 in]
                n149 = Equal?(x=w510, y=w509) -> (x = y?=w508:bool)
                n150 = case shown="True" w508 {
                  tunnel: [FALSE TRUE] -> w507
                  tunnel: w506 -> [_ w519]
                  tunnel: w505 -> [w511 w517]
                  tunnel: [w511 w516] -> w504
                  tunnel: [_ w515] -> w503
                  frame False {
                  }
                  frame True {
                    w513 = T8 []  # dblNetworkTime
                    n151 = Variant To Data(type=w513, Variant=w519) -> (data=w514:T8, error out=w515:errorcluster)  [unwired: 1 in]
                    n152 = Bundle By Name(cluster=w517, "NetworkTime"=w514) -> (w516:T2)
                  }
                }
              }
            }
            n153 = Unbundle By Name(w401) -> ("status"=w399:bool)
            n154 = Compound Arithmetic op=OR(w400, w399) -> (w398:bool)
            n155 = call <userlib>:"AddError.vi"("Severity"="Abort", "Priority"=u8 3, "ErrorArray"=w403, "error in (no error)"=w401) -> ("ErrorArray"=w402:errorcluster[])  [unwired: 6 in, 1 out]
          }
          n156 = Unregister For Events(event registration refnum=w390) -> (error out=w380:errorcluster)  [unwired: 1 in]
          n157 = call <userlib>:"AddError.vi"("Severity"="Abort", "Priority"=u8 3, "ErrorArray"=w381, "error in (no error)"=w380) -> ("ErrorArray"=w382:errorcluster[])  [unwired: 6 in, 1 out]
        }
        frame "Flag" {
          n158 = Variant To Data(type=refnum<event-registration> refnum ("Event Registration Refnum"), Variant=w522) -> (data=w520:refnum<event-registration>)  [unwired: 1 in, 1 out]
          n159 = while {
            tunnel: w531 -> [w547]
            tunnel: w520 -> [w546]
            shift-right: [w544] -> w528
            shift-left: w533 -> [w545]
            tunnel: [w539] -> w532
            shift-right: [w537] -> w529
            shift-left: w530 -> [w538]
            tunnel: w523 -> [w534]
            stop <- w540 stop-if-true
            n160 = event shown="[7] <FlagImpairBroadcasts.ReadPluginINIFilePath>: User Event" {
              selector: w546 -> [_ _ _ _ _ _ _ _ _]
              dyn-events: [_ _ _ _ _ _ _ _ _] -> w539
              timeout: 5000 -> [_ _ _ _ _ _ _ _ _]
              tunnel: w547 -> [w551 _ _ w574 _ w589 w606 w624 w641]
              tunnel: [w554 _ _ w571 _ w583 w600 w618 w635] -> w543
              tunnel: [TRUE FALSE FALSE w569 FALSE w587 w604 w622 w639] -> w542
              tunnel: w538 -> [w552 w564 w566 w568 w581 w585 w602 w620 w637]
              tunnel: [w552 w564 w566 w568 w581 w584 w601 w619 w636] -> w537
              tunnel: w534 -> [w549 _ _ _ _ _ _ _ _]
              event Timeout {
                n161 = event-data() -> ()  [unwired: 1 in, 1 out]
                n162 = xnode "Error Ring"("parameter 0"=w549, "parameter 1"="Flag" ("parameter 0"), "parameter 2"=w551) -> ("error out"=w554:errorcluster)
              }
              event User Event {
                n163 = event-data() -> ()  [unwired: 1 in, 1 out]
              }
              event User Event {
                n164 = event-data() -> ()  [unwired: 1 in, 1 out]
              }
              event User Event {
                n165 = event-data() -> ("Data"=w572:variant, "ModuleID"=w573:i32)  [unwired: 1 in]
                n166 = Equal?(x=w573, y=w574) -> (x = y?=w570:bool)
                n167 = case shown="True" w570 {
                  selector: w570 -> [w575 w576]
                  tunnel: w572 -> [_ w580]
                  tunnel: [_ w577] -> w571
                  tunnel: [w575 w576] -> w569
                  frame False {
                  }
                  frame True {
                    n168 = Variant To Data(type=T13 {"error"={"status"=FALSE, "code"=0, "source"=""}, "AdditionalInfo"=""} ("Cluster"), Variant=w580) -> (data=w578:T13)  [unwired: 1 in, 1 out]
                    n169 = Unbundle By Name(w578) -> ("error"=w577:errorcluster)
                  }
                }
              }
              event User Event {
                n170 = event-data() -> ()  [unwired: 1 in, 1 out]
              }
              event User Event {
                n171 = event-data() -> ("Data"=w586:variant, "ModuleID"=w590:i32)  [unwired: 1 in]
                n172 = Equal?(x=w590, y=w589) -> (x = y?=w588:bool)
                n173 = case shown="True" w588 {
                  selector: w588 -> [w591 w593]
                  tunnel: [w591 w593] -> w587
                  tunnel: w586 -> [_ w599]
                  tunnel: w585 -> [w592 w597]
                  tunnel: [w592 w594] -> w584
                  tunnel: [_ w596] -> w583
                  frame False {
                  }
                  frame True {
                    w598 = T10 []  # ui32FlagImpairmentArray
                    n174 = Variant To Data(type=w598, Variant=w599) -> (data=w595:T10, error out=w596:errorcluster)  [unwired: 1 in]
                    n175 = Bundle By Name(cluster=w597, "FlagImpArray"=w595) -> (w594:T2)
                  }
                }
              }
              event User Event {
                n176 = event-data() -> ("Data"=w603:variant, "ModuleID"=w607:i32)  [unwired: 1 in]
                n177 = Equal?(x=w607, y=w606) -> (x = y?=w605:bool)
                n178 = case shown="True" w605 {
                  selector: w605 -> [w608 w610]
                  tunnel: [w608 w610] -> w604
                  tunnel: w603 -> [_ w617]
                  tunnel: w602 -> [w609 w616]
                  tunnel: [w609 w615] -> w601
                  tunnel: [_ w611] -> w600
                  frame False {
                  }
                  frame True {
                    n179 = Variant To Data(type=T16 [] ("dblEventParams"), Variant=w617) -> (data=w613:T16, error out=w611:errorcluster)  [unwired: 1 in]
                    n180 = call "2DdblArrayTostrTable.vi"("dbl2DArray"=w613) -> ("strTable"=w612:string[][])  [unwired: 10 in]
                    n181 = Bundle By Name(cluster=w616, "FlagImpParams"=w612) -> (w615:T2)
                  }
                }
              }
              event User Event {
                n182 = event-data() -> ("Data"=w621:variant, "ModuleID"=w625:i32)  [unwired: 1 in]
                n183 = Equal?(x=w625, y=w624) -> (x = y?=w623:bool)
                n184 = case shown="True" w623 {
                  selector: w623 -> [w626 w629]
                  tunnel: [w626 w629] -> w622
                  tunnel: w621 -> [_ w634]
                  tunnel: w620 -> [w627 w633]
                  tunnel: [w627 w632] -> w619
                  tunnel: [_ w631] -> w618
                  frame False {
                  }
                  frame True {
                    n185 = Variant To Data(type=path "", Variant=w634) -> (data=w628:path, error out=w631:errorcluster)  [unwired: 1 in]
                    n186 = Bundle By Name(cluster=w633, "FlagImpPluginINIFilePath"=w628) -> (w632:T2)
                  }
                }
              }
              event User Event {
                n187 = event-data() -> ("Data"=w638:variant, "ModuleID"=w642:i32)  [unwired: 1 in]
                n188 = Equal?(x=w642, y=w641) -> (x = y?=w640:bool)
                n189 = case shown="True" w640 {
                  tunnel: [FALSE TRUE] -> w639
                  tunnel: w638 -> [_ _]
                  tunnel: w637 -> [w643 w646]
                  tunnel: [w643 w646] -> w636
                  tunnel: [_ errorcluster {"status"=FALSE, "code"=0, "source"=""} ("error out")] -> w635
                  frame False {
                  }
                  frame True {
                  }
                }
              }
            }
            n190 = Unbundle By Name(w543) -> ("status"=w541:bool)
            n191 = Compound Arithmetic op=OR(w542, w541) -> (w540:bool)
            n192 = call <userlib>:"AddError.vi"("Severity"="Abort", "Priority"=u8 3, "ErrorArray"=w545, "error in (no error)"=w543) -> ("ErrorArray"=w544:errorcluster[])  [unwired: 6 in, 1 out]
          }
          n193 = Unregister For Events(event registration refnum=w532) -> (error out=w526:errorcluster)  [unwired: 1 in]
          n194 = call <userlib>:"AddError.vi"("Severity"="Abort", "Priority"=u8 3, "ErrorArray"=w528, "error in (no error)"=w526) -> ("ErrorArray"=w527:errorcluster[])  [unwired: 6 in, 1 out]
        }
        frame "App" {
          n195 = Variant To Data(type=refnum<event-registration> refnum ("event registration refnum"), Variant=w649) -> (data=w650:refnum<event-registration>, error out=w648:errorcluster)  [unwired: 1 in]
          n196 = call <userlib>:"AddError.vi"("Severity"="Abort", "Priority"=u8 3, "ErrorArray"=w653, "error in (no error)"=w648) -> ("ErrorArray"=w656:errorcluster[])  [unwired: 6 in, 1 out]
          n197 = while {
            tunnel: w664 -> [w679]
            tunnel: w650 -> [w678]
            shift-right: [w676] -> w661
            shift-left: w656 -> [w677]
            tunnel: [w671] -> w665
            shift-right: [w669] -> w662
            shift-left: w663 -> [w670]
            tunnel: w652 -> [w666]
            stop <- w672 stop-if-true
            n198 = event shown="[7] <AppModuleBroadcast.OutputData>: User Event" {
              selector: w678 -> [_ _ _ _ _ _ _ _ _ _]
              dyn-events: [_ _ _ _ _ _ _ _ _ _] -> w671
              timeout: 50000 -> [_ _ _ _ _ _ _ _ _ _]
              tunnel: w679 -> [w681 _ _ w706 _ w721 w737 w751 w764 w782]
              tunnel: [w686 _ _ w703 _ w715 _ _ w758 w776] -> w675
              tunnel: [TRUE FALSE FALSE w701 FALSE w719 w735 w749 w762 w780] -> w674
              tunnel: w670 -> [w684 w696 w698 w700 w713 w717 w733 w747 w760 w778]
              tunnel: [w684 w696 w698 w700 w713 w716 w732 w746 w759 w777] -> w669
              tunnel: w666 -> [w682 _ _ _ _ _ _ _ _ _]
              event Timeout {
                n199 = event-data() -> ()  [unwired: 1 in, 1 out]
                n200 = xnode "Error Ring"("parameter 0"=w682, "parameter 1"="App" ("parameter 0"), "parameter 2"=w681) -> ("error out"=w686:errorcluster)
              }
              event User Event {
                n201 = event-data() -> ()  [unwired: 1 in, 1 out]
              }
              event User Event {
                n202 = event-data() -> ()  [unwired: 1 in, 1 out]
              }
              event User Event {
                n203 = event-data() -> ("Data"=w704:variant, "ModuleID"=w705:i32)  [unwired: 1 in]
                n204 = Equal?(x=w705, y=w706) -> (x = y?=w702:bool)
                n205 = case shown="True" w702 {
                  selector: w702 -> [w707 w708]
                  tunnel: w704 -> [_ w712]
                  tunnel: [_ w709] -> w703
                  tunnel: [w707 w708] -> w701
                  frame False {
                  }
                  frame True {
                    n206 = Variant To Data(type=T13 {"error"={"status"=FALSE, "code"=0, "source"=""}, "AdditionalInfo"=""} ("Cluster"), Variant=w712) -> (data=w710:T13)  [unwired: 1 in, 1 out]
                    n207 = Unbundle By Name(w710) -> ("error"=w709:errorcluster)
                  }
                }
              }
              event User Event {
                n208 = event-data() -> ()  [unwired: 1 in, 1 out]
              }
              event User Event {
                n209 = event-data() -> ("Data"=w718:variant, "ModuleID"=w722:i32)  [unwired: 1 in]
                n210 = Equal?(x=w722, y=w721) -> (x = y?=w720:bool)
                n211 = case shown="True" w720 {
                  tunnel: [FALSE TRUE] -> w719
                  tunnel: w718 -> [_ w728]
                  tunnel: w717 -> [w723 w730]
                  tunnel: [w723 w729] -> w716
                  tunnel: [_ w725] -> w715
                  frame False {
                  }
                  frame True {
                    n212 = Variant To Data(type=T5 [] ("ImpairReportArray"), Variant=w728) -> (data=w726:T5, error out=w725:errorcluster)  [unwired: 1 in]
                    n213 = Bundle By Name(cluster=w730, "ImpairReportArray"=w726) -> (w729:T2)
                  }
                }
              }
              event User Event {
                n214 = event-data() -> ("Data"=w734:variant, "ModuleID"=w738:i32)  [unwired: 1 in]
                n215 = Equal?(x=w738, y=w737) -> (x = y?=w736:bool)
                n216 = case shown="True" w736 {
                  tunnel: [FALSE TRUE] -> w735
                  tunnel: w734 -> [_ w741]
                  tunnel: w733 -> [w739 w743]
                  tunnel: [w739 w742] -> w732
                  frame False {
                  }
                  frame True {
                    n217 = Bundle By Name(cluster=w743, "AppConfig"=w741) -> (w742:T2)
                  }
                }
              }
              event User Event {
                n218 = event-data() -> ("Data"=w748:variant, "ModuleID"=w745:i32)  [unwired: 1 in]
                n219 = Equal?(x=w745, y=w751) -> (x = y?=w750:bool)
                n220 = case shown="True" w750 {
                  tunnel: [FALSE TRUE] -> w749
                  tunnel: w748 -> [_ w754]
                  tunnel: w747 -> [w752 w756]
                  tunnel: [w752 w755] -> w746
                  frame False {
                  }
                  frame True {
                    n221 = Bundle By Name(cluster=w756, "AppOutput"=w754) -> (w755:T2)
                  }
                }
              }
              event User Event {
                n222 = event-data() -> ("Data"=w761:variant, "ModuleID"=w765:i32)  [unwired: 1 in]
                n223 = Equal?(x=w765, y=w764) -> (x = y?=w763:bool)
                n224 = case shown="True" w763 {
                  tunnel: [FALSE TRUE] -> w762
                  tunnel: w761 -> [_ w774]
                  tunnel: w760 -> [w766 w772]
                  tunnel: [w766 w771] -> w759
                  tunnel: [_ w770] -> w758
                  frame False {
                  }
                  frame True {
                    n225 = Variant To Data(type=path "" ("AppPluginINIFilePath"), Variant=w774) -> (data=w768:path, error out=w770:errorcluster)  [unwired: 1 in]
                    n226 = Bundle By Name(cluster=w772, "AppPluginINIFilePath"=w768) -> (w771:T2)
                  }
                }
              }
              event User Event {
                n227 = event-data() -> ("Data"=w779:variant, "ModuleID"=w775:i32)  [unwired: 1 in]
                n228 = Equal?(x=w775, y=w782) -> (x = y?=w781:bool)
                n229 = case shown="True" w781 {
                  tunnel: [FALSE TRUE] -> w780
                  tunnel: w779 -> [_ _]
                  tunnel: w778 -> [w783 w786]
                  tunnel: [w783 w786] -> w777
                  tunnel: [_ errorcluster {"status"=FALSE, "code"=0, "source"=""} ("error out")] -> w776
                  frame False {
                  }
                  frame True {
                  }
                }
              }
            }
            n230 = Unbundle By Name(w675) -> ("status"=w673:bool)
            n231 = Compound Arithmetic op=OR(w674, w673) -> (w672:bool)
            n232 = call <userlib>:"AddError.vi"("Severity"="Abort", "Priority"=u8 3, "ErrorArray"=w677, "error in (no error)"=w675) -> ("ErrorArray"=w676:errorcluster[])  [unwired: 6 in, 1 out]
          }
          n233 = Unregister For Events(event registration refnum=w665) -> (error out=w659:errorcluster)  [unwired: 1 in]
          n234 = call <userlib>:"AddError.vi"("Severity"="Abort", "Priority"=u8 3, "ErrorArray"=w661, "error in (no error)"=w659) -> ("ErrorArray"=w660:errorcluster[])  [unwired: 6 in, 1 out]
        }
        frame "OutToFile" {
          n235 = Variant To Data(type=refnum<event-registration> refnum ("Event Registration Refnum 2"), Variant=w790) -> (data=w791:refnum<event-registration>, error out=w789:errorcluster)  [unwired: 1 in]
          n236 = call <userlib>:"AddError.vi"("Severity"="Abort", "Priority"=u8 3, "ErrorArray"=w793, "error in (no error)"=w789) -> ("ErrorArray"=w796:errorcluster[])  [unwired: 6 in, 1 out]
          n237 = while {
            tunnel: w804 -> [w819]
            tunnel: w791 -> [w818]
            shift-right: [w816] -> w801
            shift-left: w796 -> [w817]
            tunnel: [w811] -> w805
            shift-right: [w809] -> w802
            shift-left: w803 -> [w810]
            tunnel: w792 -> [w806]
            stop <- w812 stop-if-true
            n238 = event shown="[7] <OutputToFileBroadcast.PathToPlugin>: User Event" {
              selector: w818 -> [_ _ _ _ _ _ _ _]
              dyn-events: [_ _ _ _ _ _ _ _] -> w811
              timeout: 5000 -> [_ _ _ _ _ _ _ _]
              tunnel: w819 -> [w821 _ _ w846 _ w860 w876 w891]
              tunnel: [w826 _ _ w843 _ _ _ w885] -> w815
              tunnel: [TRUE FALSE FALSE w841 FALSE w858 w874 w889] -> w814
              tunnel: w810 -> [w824 w836 w838 w840 w853 w856 w872 w887]
              tunnel: [w824 w836 w838 w840 w853 w855 w871 w886] -> w809
              tunnel: w806 -> [w822 _ _ _ _ _ _ _]
              event Timeout {
                n239 = event-data() -> ()  [unwired: 1 in, 1 out]
                n240 = xnode "Error Ring"("parameter 0"=w822, "parameter 1"="App" ("parameter 0"), "parameter 2"=w821) -> ("error out"=w826:errorcluster)
              }
              event User Event {
                n241 = event-data() -> ()  [unwired: 1 in, 1 out]
              }
              event User Event {
                n242 = event-data() -> ()  [unwired: 1 in, 1 out]
              }
              event User Event {
                n243 = event-data() -> ("Data"=w844:variant, "ModuleID"=w845:i32)  [unwired: 1 in]
                n244 = Equal?(x=w845, y=w846) -> (x = y?=w842:bool)
                n245 = case shown="True" w842 {
                  selector: w842 -> [w847 w848]
                  tunnel: w844 -> [_ w852]
                  tunnel: [_ w849] -> w843
                  tunnel: [w847 w848] -> w841
                  frame False {
                  }
                  frame True {
                    n246 = Variant To Data(type=T13 {"error"={"status"=FALSE, "code"=0, "source"=""}, "AdditionalInfo"=""} ("Cluster"), Variant=w852) -> (data=w850:T13)  [unwired: 1 in, 1 out]
                    n247 = Unbundle By Name(w850) -> ("error"=w849:errorcluster)
                  }
                }
              }
              event User Event {
                n248 = event-data() -> ()  [unwired: 1 in, 1 out]
              }
              event User Event {
                n249 = event-data() -> ("Data"=w857:variant, "ModuleID"=w861:i32)  [unwired: 1 in]
                n250 = Equal?(x=w861, y=w860) -> (x = y?=w859:bool)
                n251 = case shown="True" w859 {
                  tunnel: [FALSE TRUE] -> w858
                  tunnel: w857 -> [_ w868]
                  tunnel: w856 -> [w862 w867]
                  tunnel: [w862 w864] -> w855
                  frame False {
                  }
                  frame True {
                    n252 = Variant To Data(type=T11 {"TIME_BASE"=1000000, "STN"="Bus_1", "IDCODE"=0, "rdoPolRect"=enum."Rectangular", "rdoFloatInt"=enum."Float", "PHUNIT"=1000000, "rdoFreqDfreq"=enum."Float", "CHNAM"=["VA", "VB", "VC", "V+", "IA", "IB", "IC", "I+"], "chkCfg2Prefix"=TRUE} ("clConfigOptions"), Variant=w868) -> (data=w865:T11)  [unwired: 1 in, 1 out]
                    n253 = Bundle By Name(cluster=w867, "clConfigOptions"=w865) -> (w864:T2)
                  }
                }
              }
              event User Event {
                n254 = event-data() -> ("Data"=w873:variant, "ModuleID"=w870:i32)  [unwired: 1 in]
                n255 = Equal?(x=w870, y=w876) -> (x = y?=w875:bool)
                n256 = case shown="True" w875 {
                  tunnel: [FALSE TRUE] -> w874
                  tunnel: w873 -> [_ w882]
                  tunnel: w872 -> [w877 w883]
                  tunnel: [w877 w879] -> w871
                  frame False {
                  }
                  frame True {
                    n257 = Variant To Data(type=path "" ("Output File Path"), Variant=w882) -> (data=w880:path)  [unwired: 1 in, 1 out]
                    n258 = Bundle By Name(cluster=w883, "Output File Path"=w880) -> (w879:T2)
                  }
                }
              }
              event User Event {
                n259 = event-data() -> ("Data"=w888:variant, "ModuleID"=w892:i32)  [unwired: 1 in]
                n260 = Equal?(x=w892, y=w891) -> (x = y?=w890:bool)
                n261 = case shown="True" w890 {
                  tunnel: [FALSE TRUE] -> w889
                  tunnel: w888 -> [_ w901]
                  tunnel: w887 -> [w893 w899]
                  tunnel: [w893 w898] -> w886
                  tunnel: [_ w897] -> w885
                  frame False {
                  }
                  frame True {
                    n262 = Variant To Data(type=path "" ("AppPluginINIFilePath"), Variant=w901) -> (data=w895:path, error out=w897:errorcluster)  [unwired: 1 in]
                    n263 = Bundle By Name(cluster=w899, "OutputToFilePluginINIFilePath"=w895) -> (w898:T2)
                  }
                }
              }
            }
            n264 = Unbundle By Name(w815) -> ("status"=w813:bool)
            n265 = Compound Arithmetic op=OR(w814, w813) -> (w812:bool)
            n266 = call <userlib>:"AddError.vi"("Severity"="Abort", "Priority"=u8 3, "ErrorArray"=w817, "error in (no error)"=w815) -> ("ErrorArray"=w816:errorcluster[])  [unwired: 6 in, 1 out]
          }
          n267 = Unregister For Events(event registration refnum=w805) -> (error out=w799:errorcluster)  [unwired: 1 in]
          n268 = call <userlib>:"AddError.vi"("Severity"="Abort", "Priority"=u8 3, "ErrorArray"=w801, "error in (no error)"=w799) -> ("ErrorArray"=w800:errorcluster[])  [unwired: 6 in, 1 out]
        }
        frame Default {
          n269 = property on="ModuleType" class="Enum (strict)"() -> ("Strings []"=w904:string[], "Value"=w903:T1)  [unwired: 2 in, 2 out]
          n270 = Index Array(array=w904, index=w903) -> (element=w902:string)
          n271 = xnode "Error Ring"("parameter 0"=w902) -> ("error out"=w909:errorcluster)
          n272 = call <userlib>:"AddError.vi"("Severity"="Abort", "Priority"=u8 3, "ErrorArray"=w910, "error in (no error)"=w909) -> ("ErrorArray"=w908:errorcluster[])  [unwired: 6 in, 1 out]
        }
      }
    }
  }
  "Error Out" <- w15
  "clBusData Out" <- w13
